vi "Obtain.vi"(8 "error in (no error)":errorcluster, 11 "Connection":T1={"IP Address"="localhost", "Port"=50007, "ConnectTMO"=1000}) -> (0 "error out":errorcluster, 3 "TcpRouter-Client out":refnum<class "TcpRouter-Client.lvclass">)   [LabVIEW 2020, in "CSM-TCP-Router.lvlib" / "TcpRouter-Client.lvclass"]
uses:
  TcpRouter-Client.lvclass
  Def-TCP-Router REQ-REP.ctl
  Def-TCP-Router PUB-SUB.ctl
  Def-TCP-Router Status Data.ctl
  Def-TCP-Router ASYNC-RESP.ctl
  Def-TCP-Router Async-Resp Data.ctl
  TcpRouter-Client.lvclass/TcpRouter-Client.ctl
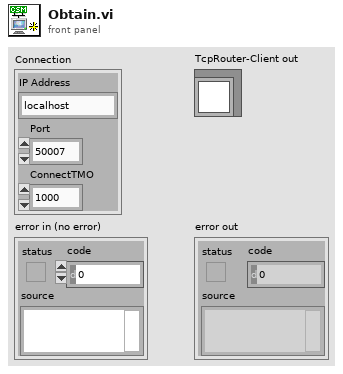
[diagram p1: front panel]
types:
  T1 = cluster{"IP Address":string, "Port":u16, "ConnectTMO":i32}
  T2 = typedef "CSM-TCP-Router.lvlib/TcpRouter-Client.lvclass/Def-TCP-Router ASYNC-RESP.ctl" = cluster{"Async-Resp":refnum<k5>, "RespQueue":refnum<queue>, "RespEvent":refnum<user-event>}
  T3 = typedef "CSM-TCP-Router.lvlib/TcpRouter-Client.lvclass/Def-TCP-Router PUB-SUB.ctl" = cluster{"STATUS":refnum<k5>, "StatusQueue":refnum<queue>}
  T4 = typedef "CSM-TCP-Router.lvlib/TcpRouter-Client.lvclass/Def-TCP-Router REQ-REP.ctl" = cluster{"REQ-REP":refnum<k5>}
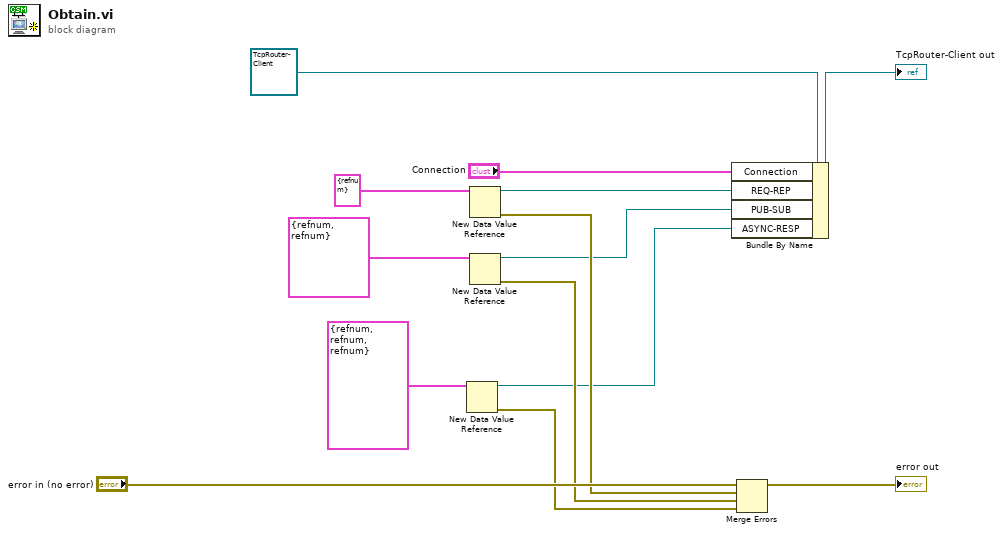
[diagram p0: block diagram]
diagram:
  n1 = New Data Value Reference(data value=T2 {"Async-Resp"=refnum, "RespQueue"=refnum, "RespEvent"=refnum} ("TCP-Router Client Data")) -> (data value reference=w2:refnum<data-value>, error out=w1:errorcluster)  [unwired: 1 in]
  n2 = New Data Value Reference(data value=T4 {"REQ-REP"=refnum} ("TCP-Router Client Data")) -> (data value reference=w10:refnum<data-value>, error out=w8:errorcluster)  [unwired: 1 in]
  n3 = New Data Value Reference(data value=T3 {"STATUS"=refnum, "StatusQueue"=refnum} ("TCP-Router Client Data")) -> (data value reference=w5:refnum<data-value>, error out=w4:errorcluster)  [unwired: 1 in]
  n4 = Bundle By Name(cluster=refnum<class "TcpRouter-Client.lvclass"> refnum ("TcpRouter-Client in"), "Connection"="Connection", "REQ-REP"=w10, "PUB-SUB"=w5, "ASYNC-RESP"=w2) -> (→"TcpRouter-Client out":refnum<class "TcpRouter-Client.lvclass">)
  n5 = Merge Errors("error in (no error)", w8, w4, w1) -> (→"error out":errorcluster)
